vi "Assert Collection Not Contains.vi"(5 "Expected":variant, 7 "Message (\"\")":string, 8 "error in (no error)":errorcluster, 10 "Collection":variant) -> (0 "error out":errorcluster)   [LabVIEW 2017, in "Transparent Assertions.lvlib"]
doc: "Asserts that a collection (array, set, or map) does not contain the expected value. Returns an error if the assertion fails, and optionally appends a custom message to the error.\n\nFor maps, the expected value is compared against the values in the map."
uses:
  Transparent Assertions.lvlib
  LogicalNot/LogicalNot.lvclass
  Collection Contains/Collection Contains.lvclass
  C:/Users/pasca/Projects/Home/TransparentAssertions/src/Transparent Assertions/Constraints/Constraint/Constraint.lvclass
  UnaryOperator/UnaryOperator.lvclass
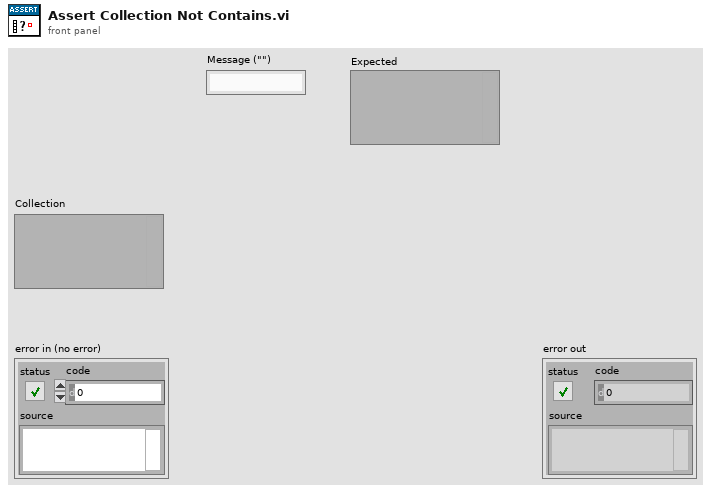
[diagram p1: front panel]
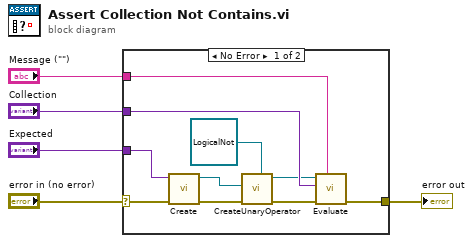
[diagram p0: block diagram]
diagram:
  n1 = case shown="No Error" "error in (no error)" {
    selector: "error in (no error)" -> [w10 w16]
    tunnel: [w15 w16] -> w5
    tunnel: "Collection" -> [w14 _]
    tunnel: "Message (\"\")" -> [w13 _]
    tunnel: "Expected" -> [w12 _]
    frame No Error {
      n2 = call "Create.vi"("error in (no error)"=w10, "Item"=w12) -> ("error out"=w11:errorcluster, "Collection Contains"=w8:refnum<class "Collection Contains.lvclass">)  [unwired: 8 in]
      n3 = call-dynamic "CreateUnaryOperator.vi"("UnaryOperator In"=refnum<class "LogicalNot.lvclass"> refnum ("Transparent Assertions.lvlib:Constraints.lvlib:LogicalNot.lvclass"), "error in (no error)"=w11, "Constraint"=w8) -> ("error out"=w9:errorcluster, "UnaryOperator"=w7:refnum<class "UnaryOperator.lvclass">)  [unwired: 7 in]
      n4 = call-dynamic "Evaluate.vi"("Message (\"\")"=w13, "error in (no error)"=w9, "Actual"=w14, "Constraint in"=w7) -> ("error out"=w15:errorcluster)  [unwired: 6 in, 1 out]
    }
    frame Error {
    }
  }
  "error out" <- w5
